vi "gun_lock_store.vi"(10 "data_store_mode":enum16{"Set", "Get"}(ring), 11 "Lock":bool) -> (3 "Lock":bool)   [LabVIEW 2011]
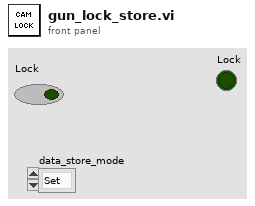
[diagram p1: front panel]
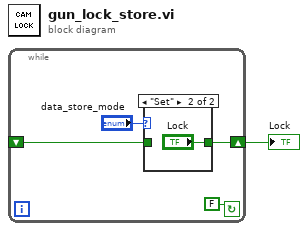
[diagram p0: block diagram]
diagram:
  n1 = while {
    shift-right: [w3] -> w1
    shift-left: _ -> [w2]
    stop <- FALSE continue-if-true
    n2 = case shown="\"Set\"" "data_store_mode" {
      tunnel: [w6 "Lock"] -> w3
      tunnel: w2 -> [w6 _]
      frame Default {
      }
      frame "Set" {
      }
    }
  }
  "Lock" <- w1
